vi "Read Cells.vi"(8 "error in (no error)":errorcluster, 11 "CRDS in":refnum<class "CRDS.lvclass">) -> (0 "error out":errorcluster, 2 "Cells":refnum<class "CRDS Cell.lvclass">[](array[class]), 3 "CRDS out":refnum<class "CRDS.lvclass">)   [LabVIEW 2015, in "CRDS.lvclass"]
uses:
  CRDS.lvclass
  Cell/CRDS Cell.lvclass
  CRDS.lvclass/CRDS.ctl
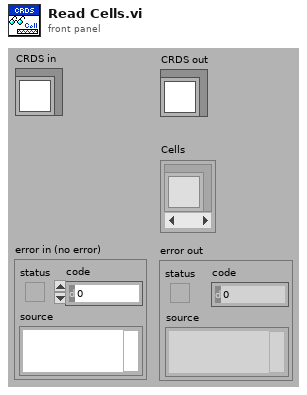
[diagram p1: front panel]
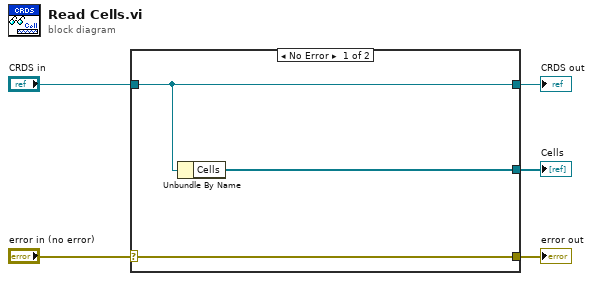
[diagram p0: block diagram]
diagram:
  n1 = case shown="No Error" "error in (no error)" {
    selector: "error in (no error)" -> [w8 w9]
    tunnel: [w8 w9] -> w4
    tunnel: [w7 w10] -> w2
    tunnel: "CRDS in" -> [w7 w10]
    tunnel: [w6 _] -> w1
    frame No Error {
      n2 = Unbundle By Name(w7) -> ("Cells"=w6:refnum<class "CRDS Cell.lvclass">[])
    }
    frame Error {
    }
  }
  "error out" <- w4
  "CRDS out" <- w2
  "Cells" <- w1
